vi "Read Hardware Settings.vi"(8 "error in (no error)":errorcluster, 11 "Boot Loader in":refnum<class "Boot Loader.lvclass">) -> (0 "error out":errorcluster, 2 "Hardware Settings":T1, 3 "Boot Loader out":refnum<class "Boot Loader.lvclass">)   [LabVIEW 2015, in "Boot Loader.lvclass"]
uses:
  Boot Loader.lvclass
  Typedefs/Hardware Settings.ctl
  Typedefs/Actuator Types.ctl
  Typedefs/Cylinder Types.ctl
  Settings/Settings.lvclass
  Typedefs/FAMT Typedefs.lvlib
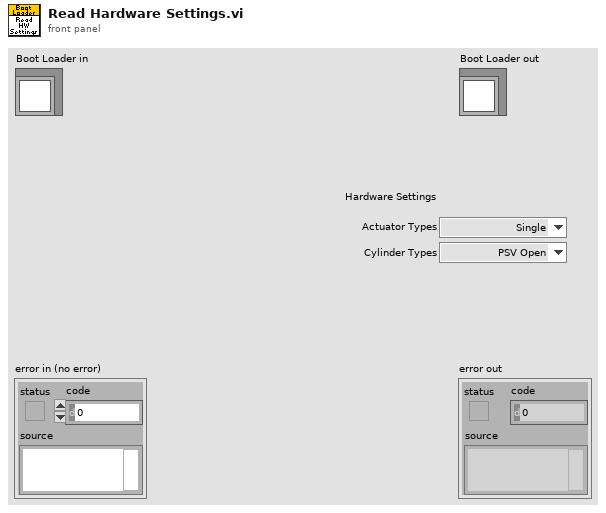
[diagram p1: front panel]
types:
  T1 = typedef "FAMT Typedefs.lvlib/Hardware Settings.ctl" = cluster{"Actuator Types":T2, "Cylinder Types":T3}
  T2 = typedef "FAMT Typedefs.lvlib/Actuator Types.ctl" = enum16{"Single", "Dual"}
  T3 = typedef "FAMT Typedefs.lvlib/Cylinder Types.ctl" = enum16{"PSV Open", "PSV Closed", "TV Open", "TV Closed", "Closed"}
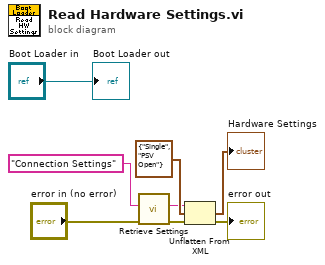
[diagram p0: block diagram]
diagram:
  n1 = call "Retrieve Settings.vi"("error in (no error)"="error in (no error)", "configName"="Connection Settings") -> ("error out"=w2:errorcluster, "xmlConfig"=w6:string)  [unwired: 7 in, 1 out]
  n2 = Unflatten From XML(xml string=w6, type=T1 {"Actuator Types"=enum."Single", "Cylinder Types"=enum."PSV Open"} ("Hardware Settings"), error in (no error)=w2) -> (value=→"Hardware Settings":T1, error out=→"error out":errorcluster)
  "Boot Loader out" <- "Boot Loader in"
